vi "rsidr_core_global.vi"() -> ()   [LabVIEW 2020, in "Rohde&Schwarz CMWXP NR FR1 Measurement.lvlib"] (continued)
 "Flags"=0, "Help"="Put a help here"}, {"Level"=3, "Class Only"=FALSE, "Identifier"="RSCMWXPNRFR1M_ATTR_MULTI_EVAL_MEAS_TRIGGER_SOURCE", "Descriptive Name"="Multi Eval Meas Trigger Source", "Data Type"=enum."ViString", "Command"="TRIG:NRS:MEAS{instance}:MEV:SOUR", "Access"=enum."Read/Write", "Range Table"="", "Read Callback"="", "Write Callback"="", "Range Callback"="", "Check Callback"="", "Rngtable Callback"="", "Coerce Callback"="", "Supported Models"="", "Instrument Options"="", "Check Status Callback"="", "Flags"=0, "Help"="Selects the source of the trigger events. Some values are always available. They are listed below. Depending on the installed options, additional values are available. You can query a list of all supported values via TRIGger:...:CATalog:SOURce?.\n\nAvailable Repeated Capabilities:\ninstance: i0, i1, i2, i3, i4, i5, i6, i7, i8, i9, i10, i11, i12, i13, i14, i15, i16, i17, i18, i19, i20, i21, i22, i23, i24, i25, i26, i27, i28, i29, i30, i31, i32\r\n\nRemote-control command(s):\nTRIGger:NRSub:MEAS<i>:MEValuation:SOURce"}, {"Level"=3, "Class Only"=FALSE, "Identifier"="RSCMWXPNRFR1M_ATTR_MULTI_EVAL_MEAS_TRIGGER_SOURCE_CATALOG", "Descriptive Name"="Multi Eval Meas Trigger Source Catalog", "Data Type"=enum."RawString", "Command"="TRIG:NRS:MEAS{instance}:MEV:CAT:SOUR?", "Access"=enum."Read Only", "Range Table"="", "Read Callback"="", "Write Callback"="", "Range Callback"="", "Check Callback"="", "Rngtable Callback"="", "Coerce Callback"="", "Supported Models"="", "Instrument Options"="", "Check Status Callback"="", "Flags"=0, "Help"="Lists all trigger source values that can be set using TRIGger:NRSub:MEAS<i>:MEValuation:SOURce.\n\nAvailable Repeated Capabilities:\ninstance: i0, i1, i2, i3, i4, i5, i6, i7, i8, i9, i10, i11, i12, i13, i14, i15, i16, i17, i18, i19, i20, i21, i22, i23, i24, i25, i26, i27, i28, i29, i30, i31, i32\r\n\nRemote-control command(s):\nTRIGger:NRSub:MEAS<i>:MEValuation:CATalog:SOURce?"}, {"Level"=3, "Class Only"=FALSE, "Identifier"="RSCMWXPNRFR1M_ATTR_MULTI_EVAL_MEAS_TRIGGER_SLOPE", "Descriptive Name"="Multi Eval Meas Trigger Slope", "Data Type"=enum."ViInt32", "Command"="TRIG:NRS:MEAS{instance}:MEV:SLOP", "Access"=enum."Read/Write", "Range Table"="rsCmwxpNrFr1M_rngTrigSlope", "Read Callback"="", "Write Callback"="", "Range Callback"="", "Check Callback"="", "Rngtable Callback"="", "Coerce Callback"="", "Supported Models"="", "Instrument Options"="", "Check Status Callback"="", "Flags"=0, "Help"="Qualifies whether the trigger event is generated at the rising or at the falling edge of the trigger pulse (valid for external and power trigger sources).\n\nAvailable Repeated Capabilities:\ninstance: i0, i1, i2, i3, i4, i5, i6, i7, i8, i9, i10, i11, i12, i13, i14, i15, i16, i17, i18, i19, i20, i21, i22, i23, i24, i25, i26, i27, i28, i29, i30, i31, i32\r\n\nRemote-control command(s):\nTRIGger:NRSub:MEAS<i>:MEValuation:SLOPe"}, {"Level"=3, "Class Only"=FALSE, "Identifier"="RSCMWXPNRFR1M_ATTR_MULTI_EVAL_MEAS_TRIGGER_THRESHOLD", "Descriptive Name"="Multi Eval Meas Trigger Threshold", "Data Type"=enum."ViReal64", "Command"="TRIG:NRS:MEAS{instance}:MEV:THR", "Access"=enum."Read/Write", "Range Table"="rsCmwxpNrFr1M_rngTrigThreshold", "Read Callback"="", "Write Callback"="", "Range Callback"="", "Check Callback"="", "Rngtable Callback"="", "Coerce Callback"="", "Supported Models"="", "Instrument Options"="", "Check Status Callback"="", "Flags"=0, "Help"="Defines the trigger threshold for power trigger sources.\n\nAvailable Repeated Capabilities:\ninstance: i0, i1, i2, i3, i4, i5, i6, i7, i8, i9, i10, i11, i12, i13, i14, i15, i16, i17, i18, i19, i20, i21, i22, i23, i24, i25, i26, i27, i28, i29, i30, i31, i32\r\n\nRemote-control command(s):\nTRIGger:NRSub:MEAS<i>:MEValuation:THReshold"}, {"Level"=3, "Class Only"=FALSE, "Identifier"="RSCMWXPNRFR1M_ATTR_MULTI_EVAL_MEAS_TRIGGER_DELAY", "Descriptive Name"="Multi Eval Meas Trigger Delay", "Data Type"=enum."ViReal64", "Command"="TRIG:NRS:MEAS{instance}:MEV:DEL", "Access"=enum."Read/Write", "Range Table"="rsCmwxpNrFr1M_rngMultiEvalMeasurementTriggerDelay", "Read Callback"="", "Write Callback"="", "Range Callback"="", "Check Callback"="", "Rngtable Callback"="", "Coerce Callback"="", "Supported Models"="", "Instrument Options"="", "Check Status Callback"="", "Flags"=0, "Help"="Defines a time delaying the start of the measurement relative to the trigger event. This setting has no influence on free run measurements.\n\nAvailable Repeated Capabilities:\ninstance: i0, i1, i2, i3, i4, i5, i6, i7, i8, i9, i10, i11, i12, i13, i14, i15, i16, i17, i18, i19, i20, i21, i22, i23, i24, i25, i26, i27, i28, i29, i30, i31, i32\r\n\nRemote-control command(s):\nTRIGger:NRSub:MEAS<i>:MEValuation:DELay"}, {"Level"=3, "Class Only"=FALSE, "Identifier"="RSCMWXPNRFR1M_ATTR_MULTI_EVAL_MEAS_TRIGGER_TIMEOUT_ENABLED", "Descriptive Name"="Multi Eval Meas Trigger Timeout Enabled", "Data Type"=enum."ViBoolean", "Command"="TRIG:NRS:MEAS{instance}:MEV:TOUT", "Access"=enum."Read/Write", "Range Table"="", "Read Callback"="", "Write Callback"="", "Range Callback"="", "Check Callback"="", "Rngtable Callback"="", "Coerce Callback"="", "Supported Models"="", "Instrument Options"="", "Check Status Callback"="", "Flags"=0, "Help"="Selects the maximum time that the measurement waits for a trigger event before it stops in remote control mode or indicates a trigger timeout in manual operation mode. This setting has no influence on Free Run measurements.\n\nAvailable Repeated Capabilities:\ninstance: i0, i1, i2, i3, i4, i5, i6, i7, i8, i9, i10, i11, i12, i13, i14, i15, i16, i17, i18, i19, i20, i21, i22, i23, i24, i25, i26, i27, i28, i29, i30, i31, i32\r\n\nRemote-control command(s):\nTRIGger:NRSub:MEAS<i>:MEValuation:TOUT"}, {"Level"=3, "Class Only"=FALSE, "Identifier"="RSCMWXPNRFR1M_ATTR_MULTI_EVAL_MEAS_TRIGGER_TIMEOUT", "Descriptive Name"="Multi Eval Meas Trigger Timeout", "Data Type"=enum."ViReal64", "Command"="TRIG:NRS:MEAS{instance}:MEV:TOUT", "Access"=enum."Read/Write", "Range Table"="rsCmwxpNrFr1M_rngTriggerTimeout", "Read Callback"="", "Write Callback"="", "Range Callback"="", "Check Callback"="", "Rngtable Callback"="", "Coerce Callback"="", "Supported Models"="", "Instrument Options"="", "Check Status Callback"="", "Flags"=0, "Help"="Selects the maximum time that the measurement waits for a trigger event before it stops in remote control mode or indicates a trigger timeout in manual operation mode. This setting has no influence on Free Run measurements.\n\nAvailable Repeated Capabilities:\ninstance: i0, i1, i2, i3, i4, i5, i6, i7, i8, i9, i10, i11, i12, i13, i14, i15, i16, i17, i18, i19, i20, i21, i22, i23, i24, i25, i26, i27, i28, i29, i30, i31, i32\r\n\nRemote-control command(s):\nTRIGger:NRSub:MEAS<i>:MEValuation:TOUT"}, {"Level"=3, "Class Only"=FALSE, "Identifier"="RSCMWXPNRFR1M_ATTR_MULTI_EVAL_MEAS_MINIMUM_TRIGGER_GAP", "Descriptive Name"="Multi Eval Meas Minimum Trigger Gap", "Data Type"=enum."ViReal64", "Command"="TRIG:NRS:MEAS{instance}:MEV:MGAP", "Access"=enum."Read/Write", "Range Table"="rsCmwxpNrFr1M_rngMinimumTriggerGap", "Read Callback"="", "Write Callback"="", "Range Callback"="", "Check Callback"="", "Rngtable Callback"="", "Coerce Callback"="", "Supported Models"="", "Instrument Options"="", "Check Status Callback"="", "Flags"=0, "Help"="Sets a minimum time during which the IF signal must be below the trigger threshold before the trigger is armed so that an IF power trigger event can be generated.\n\nAvailable Repeated Capabilities:\ninstance: i0, i1, i2, i3, i4, i5, i6, i7, i8, i9, i10, i11, i12, i13, i14, i15, i16, i17, i18, i19, i20, i21, i22, i23, i24, i25, i26, i27, i28, i29, i30, i31, i32\r\n\nRemote-control command(s):\nTRIGger:NRSub:MEAS<i>:MEValuation:MGAP"}, {"Level"=3, "Class Only"=FALSE, "Identifier"="RSCMWXPNRFR1M_ATTR_MULTI_EVAL_MEAS_TRIGGER_SYNC_MODE", "Descriptive Name"="Multi Eval Meas Trigger Sync Mode", "Data Type"=enum."ViInt32", "Command"="TRIG:NRS:MEAS{instance}:MEV:SMOD", "Access"=enum."Read/Write", "Range Table"="rsCmwxpNrFr1M_rngTriggerSyncMode", "Read Callback"="", "Write Callback"="", "Range Callback"="", "Check Callback"="", "Rngtable Callback"="", "Coerce Callback"="", "Supported Models"="", "Instrument Options"="", "Check Status Callback"="", "Flags"=0, "Help"="Selects the size of the search window for synchronization - normal or enhanced.\n\nAvailable Repeated Capabilities:\ninstance: i0, i1, i2, i3, i4, i5, i6, i7, i8, i9, i10, i11, i12, i13, i14, i15, i16, i17, i18, i19, i20, i21, i22, i23, i24, i25, i26, i27, i28, i29, i30, i31, i32\r\n\nRemote-control command(s):\nTRIGger:NRSub:MEAS<i>:MEValuation:SMODe"}, {"Level"=3, "Class Only"=FALSE, "Identifier"="RSCMWXPNRFR1M_ATTR_MULTI_EVAL_MEAS_TRIGGER_LIST_MODE", "Descriptive Name"="Multi Eval Meas Trigger List Mode", "Data Type"=enum."ViInt32", "Command"="TRIG:NRS:MEAS{instance}:MEV:LIST:MODE", "Access"=enum."Read/Write", "Range Table"="rsCmwxpNrFr1M_rngTriggerListMode", "Read Callback"="", "Write Callback"="", "Range Callback"="", "Check Callback"="", "Rngtable Callback"="", "Coerce Callback"="", "Supported Models"="", "Instrument Options"="", "Check Status Callback"="", "Flags"=0, "Help"="Specifies the trigger mode for list mode measurements. For configuration of retrigger flags, see CONFigure:NRSub:MEAS<i>:LIST:SEGMent<no>:SETup.\n\nAvailable Repeated Capabilities:\ninstance: i0, i1, i2, i3, i4, i5, i6, i7, i8, i9, i10, i11, i12, i13, i14, i15, i16, i17, i18, i19, i20, i21, i22, i23, i24, i25, i26, i27, i28, i29, i30, i31, i32\r\n\nRemote-control command(s):\nTRIGger:NRSub:MEAS<i>:MEValuation:LIST:MODE"}, {"Level"=2, "Class Only"=TRUE, "Identifier"="", "Descriptive Name"="Limits", "Data Type"=enum."ViInt32", "Command"="", "Access"=enum."Read Only", "Range Table"="", "Read Callback"="", "Write Callback"="", "Range Callback"="", "Check Callback"="", "Rngtable Callback"="", "Coerce Callback"="", "Supported Models"="", "Instrument Options"="", "Check Status Callback"="", "Flags"=0, "Help"="Multi Evaluation measurement limits attributes."}, {"Level"=3, "Class Only"=TRUE, "Identifier"="", "Descriptive Name"="Modulation", "Data Type"=enum."ViInt32", "Command"="", "Access"=enum."Read Only", "Range Table"="", "Read Callback"="", "Write Callback"="", "Range Callback"="", "Check Callback"="", "Rngtable Callback"="", "Coerce Callback"="", "Supported Models"="", "Instrument Options"="", "Check Status Callback"="", "Flags"=0, "Help"="Contains attributes for selected modulation."}, {"Level"=4, "Class Only"=TRUE, "Identifier"="", "Descriptive Name"="Pi/2-BPSK", "Data Type"=enum."ViInt32", "Command"="", "Access"=enum."Read Only", "Range Table"="", "Read Callback"="", "Write Callback"="", "Range Callback"="", "Check Callback"="", "Rngtable Callback"="", "Coerce Callback"="", "Supported Models"="", "Instrument Options"="", "Check Status Callback"="", "Flags"=0, "Help"="Define limits for results which characterize the modulation accuracy of signals with modulation scheme Pi/2-BPSK."}, {"Level"=5, "Class Only"=FALSE, "Identifier"="RSCMWXPNRFR1M_ATTR_MULTI_EVAL_MEAS_LIMIT_PI_2_EVM", "Descriptive Name"="Multi Eval Meas Limit Pi/2 BPSK EVM", "Data Type"=enum."RawString", "Command"="CONF:NRS:MEAS{instance}:MEV:LIM:PHBP:EVM", "Access"=enum."Read/Write", "Range Table"="", "Read Callback"="", "Write Callback"="", "Range Callback"="", "Check Callback"="", "Rngtable Callback"="", "Coerce Callback"="", "Supported Models"="", "Instrument Options"="", "Check Status Callback"="", "Flags"=0, "Help"="Defines upper limits for the RMS and peak values of the error vector magnitude (EVM) for Pi/2-BPSK.\n\nSyntax:\nCONFigure:NRSub:MEAS<i>:MEValuation:LIMit:PHBPsk:EVMagnitude <RMS>, <Peak>\n\n<RMS>\nnumeric | ON | OFF\nValid Values:\n0 % to 100 %\n  \n<Peak>\nnumeric | ON | OFF\nValid Values:\n0 % to 100 %\n\nAvailable Repeated Capabilities:\ninstance: i0, i1, i2, i3, i4, i5, i6, i7, i8, i9, i10, i11, i12, i13, i14, i15, i16, i17, i18, i19, i20, i21, i22, i23, i24, i25, i26, i27, i28, i29, i30, i31, i32\r\n\nRemote-control command(s):\nCONFigure:NRSub:MEAS<i>:MEValuation:LIMit:PHBPsk:EVMagnitude"}, {"Level"=5, "Class Only"=FALSE, "Identifier"="RSCMWXPNRFR1M_ATTR_MULTI_EVAL_MEAS_LIMIT_PI_2_MERR", "Descriptive Name"="Multi Eval Meas Limit Pi/2 BPSK MERR", "Data Type"=enum."RawString", "Command"="CONF:NRS:MEAS{instance}:MEV:LIM:PHBP:MERR", "Access"=enum."Read/Write", "Range Table"="", "Read Callback"="", "Write Callback"="", "Range Callback"="", "Check Callback"="", "Rngtable Callback"="", "Coerce Callback"="", "Supported Models"="", "Instrument Options"="", "Check Status Callback"="", "Flags"=0, "Help"="Defines upper limits for the RMS and peak values of the magnitude error for Pi/2-BPSK.\n\nSyntax:\nCONFigure:NRSub:MEAS<i>:MEValuation:LIMit:PHBPsk:MERRor <RMS>, <Peak>\n\n<RMS>\nnumeric | ON | OFF\nValid Values:\n0 % to 100 %\n  \n<Peak>\nnumeric | ON | OFF\nValid Values:\n0 % to 100 %\n\nAvailable Repeated Capabilities:\ninstance: i0, i1, i2, i3, i4, i5, i6, i7, i8, i9, i10, i11, i12, i13, i14, i15, i16, i17, i18, i19, i20, i21, i22, i23, i24, i25, i26, i27, i28, i29, i30, i31, i32\r\n\nRemote-control command(s):\nCONFigure:NRSub:MEAS<i>:MEValuation:LIMit:PHBPsk:MERRor"}, {"Level"=5, "Class Only"=FALSE, "Identifier"="RSCMWXPNRFR1M_ATTR_MULTI_EVAL_MEAS_LIMIT_PI_2_PERR", "Descriptive Name"="Multi Eval Meas Limit Pi/2 BPSK PERR", "Data Type"=enum."RawString", "Command"="CONF:NRS:MEAS{instance}:MEV:LIM:PHBP:PERR", "Access"=enum."Read/Write", "Range Table"="", "Read Callback"="", "Write Callback"="", "Range Callback"="", "Check Callback"="", "Rngtable Callback"="", "Coerce Callback"="", "Supported Models"="", "Instrument Options"="", "Check Status Callback"="", "Flags"=0, "Help"="Defines symmetric limits for the RMS and peak values of the phase error for Pi/2-BPSK. The limit check fails if the absolute value of the measured phase error exceeds the specified values.\n\nSyntax:\nCONFigure:NRSub:MEAS<i>:MEValuation:LIMit:PHBPsk:PERRor <RMS>, <Peak>\n\n<RMS>\nnumeric | ON | OFF\nValid Values:\n0 deg to 180 deg\n  \n<Peak>\nnumeric | ON | OFF\nValid Values:\n0 deg to 180 deg\n\nAvailable Repeated Capabilities:\ninstance: i0, i1, i2, i3, i4, i5, i6, i7, i8, i9, i10, i11, i12, i13, i14, i15, i16, i17, i18, i19, i20, i21, i22, i23, i24, i25, i26, i27, i28, i29, i30, i31, i32\r\n\nRemote-control command(s):\nCONFigure:NRSub:MEAS<i>:MEValuation:LIMit:PHBPsk:PERRor"}, {"Level"=5, "Class Only"=FALSE, "Identifier"="RSCMWXPNRFR1M_ATTR_MULTI_EVAL_MEAS_LIMIT_PI_2_FERR_ENABLED", "Descriptive Name"="Multi Eval Meas Limit Pi/2 BPSK FERR Enabled", "Data Type"=enum."ViBoolean", "Command"="CONF:NRS:MEAS{instance}:MEV:LIM:PHBP:FERR", "Access"=enum."Read/Write", "Range Table"="", "Read Callback"="", "Write Callback"="", "Range Callback"="", "Check Callback"="", "Rngtable Callback"="", "Coerce Callback"="", "Supported Models"="", "Instrument Options"="", "Check Status Callback"="", "Flags"=0, "Help"="Defines an upper limit for the carrier frequency error (Pi/2-BPSK modulation).\n\nAvailable Repeated Capabilities:\ninstance: i0, i1, i2, i3, i4, i5, i6, i7, i8, i9, i10, i11, i12, i13, i14, i15, i16, i17, i18, i19, i20, i21, i22, i23, i24, i25, i26, i27, i28, i29, i30, i31, i32\r\n\nRemote-control command(s):\nCONFigure:NRSub:MEAS<i>:MEValuation:LIMit:PHBPsk:FERRor"}, {"Level"=5, "Class Only"=FALSE, "Identifier"="RSCMWXPNRFR1M_ATTR_MULTI_EVAL_MEAS_LIMIT_PI_2_FERR", "Descriptive Name"="Multi Eval Meas Limit Pi/2 BPSK FERR", "Data Type"=enum."ViReal64", "Command"="CONF:NRS:MEAS{instance}:MEV:LIM:PHBP:FERR", "Access"=enum."Read/Write", "Range Table"="rsCmwxpNrFr1M_rngFERR", "Read Callback"="", "Write Callback"="", "Range Callback"="", "Check Callback"="", "Rngtable Callback"="", "Coerce Callback"="", "Supported Models"="", "Instrument Options"="", "Check Status Callback"="", "Flags"=0, "Help"="Defines an upper limit for the carrier frequency error (Pi/2-BPSK modulation).\n\nAvailable Repeated Capabilities:\ninstance: i0, i1, i2, i3, i4, i5, i6, i7, i8, i9, i10, i11, i12, i13, i14, i15, i16, i17, i18, i19, i20, i21, i22, i23, i24, i25, i26, i27, i28, i29, i30, i31, i32\r\n\nRemote-control command(s):\nCONFigure:NRSub:MEAS<i>:MEValuation:LIMit:PHBPsk:FERRor"}, {"Level"=5, "Class Only"=FALSE, "Identifier"="RSCMWXPNRFR1M_ATTR_MULTI_EVAL_MEAS_LIMIT_PI_2_IQ_OFFSET", "Descriptive Name"="Multi Eval Meas Limit Pi/2 BPSK IQ Offset", "Data Type"=enum."RawString", "Command"="CONF:NRS:MEAS{instance}:MEV:LIM:PHBP:IQOF", "Access"=enum."Read/Write", "Range Table"="", "Read Callback"="", "Write Callback"="", "Range Callback"="", "Check Callback"="", "Rngtable Callback"="", "Coerce Callback"="", "Supported Models"="", "Instrument Options"="", "Check Status Callback"="", "Flags"=0, "Help"="Defines upper limits for the I/Q origin offset (Pi/2-BPSK modulation). Four different I/Q origin offset limits can be set for four TX power ranges.\n\nSyntax:\nCONFigure:NRSub:MEAS<i>:MEValuation:LIMit:PHBPsk:IQOFfset <Enable>, <Offset0>, <Offset1>,<Offset2>,<Offset3>\n\n<Enable>\nValid Values:\nOFF: disables the limit check\nON: enables the limit check\n\n<Offset0>\nI/Q origin offset limit for TX power > 10 dBm\nnumeric\nValid Values: -256 dBc to 256 dBc\n\n<Offset1>\nI/Q origin offset limit for TX power > 0 dBm\nnumeric\nValid Values: -256 dBc to 256 dBc\n\n<Offset2>\nI/Q origin offset limit for TX power > -30 dBm\nnumeric\nValid Values: -256 dBc to 256 dBc\n\n<Offset3>\nI/Q origin offset limit for TX power > -40 dBm\nnumeric\nValid Values: -256 dBc to 256 dBc\n\nAvailable Repeated Capabilities:\ninstance: i0, i1, i2, i3, i4, i5, i6, i7, i8, i9, i10, i11, i12, i13, i14, i15, i16, i17, i18, i19, i20, i21, i22, i23, i24, i25, i26, i27, i28, i29, i30, i31, i32\r\n\nRemote-control command(s):\nCONFigure:NRSub:MEAS<i>:MEValuation:LIMit:PHBPsk:IQOFfset"}, {"Level"=5, "Class Only"=FALSE, "Identifier"="RSCMWXPNRFR1M_ATTR_MULTI_EVAL_MEAS_LIMIT_PI_2_INBAND_EMISSION", "Descriptive Name"="Multi Eval Meas Limit Pi/2 BPSK Inband Emission", "Data Type"=enum."RawString", "Command"="CONF:NRS:MEAS{instance}:MEV:LIM:PHBP:IBE", "Access"=enum."Read/Write", "Range Table"="", "Read Callback"="", "Write Callback"="", "Range Callback"="", "Check Callback"="", "Rngtable Callback"="", "Coerce Callback"="", "Supported Models"="", "Instrument Options"="", "Check Status Callback"="", "Flags"=0, "Help"="Defines parameters used for calculation of an upper limit for the inband emission (Pi/2-BPSK modulation), see 'Inband Emissions Limits'.\n\nSyntax:\nCONFigure:NRSub:MEAS<i>:MEValuation:LIMit:PHBPsk:IBE <Enable>, <Minimum>, <EVM>, <RBPower>, <IQImageLesser>, <IQImageGreater>\n\n<Enable>\nValid Values:\nOFF: disables the limit check\nON: enables the limit check\n\n<Minimum>\nnumeric\nValid Values: -256 dB to 256 dB\n\n<EVM>\nnumeric\nValid Values: 0 % to 100 %\n\n<RBPower>\nnumeric\nValid Values: -256 dBm to 256 dBm\n\n<IQImageLesser>\nIQ image for low TX power range\nnumeric\nValid Values: -256 dB to 256 dB\n \n<IQImageGreater>\nIQ image for high TX power range\nnumeric\nValid Values: -256 dB  to  256 dB\n\nAvailable Repeated Capabilities:\ninstance: i0, i1, i2, i3, i4, i5, i6, i7, i8, i9, i10, i11, i12, i13, i14, i15, i16, i17, i18, i19, i20, i21, i22, i23, i24, i25, i26, i27, i28, i29, i30, i31, i32\r\n\nRemote-control command(s):\nCONFigure:NRSub:MEAS<i>:MEValuation:LIMit:PHBPsk:IBE"}, {"Level"=5, "Class Only"=FALSE, "Identifier"="RSCMWXPNRFR1M_ATTR_MULTI_EVAL_MEAS_LIMIT_PI_2_INBAND_EMISSION_IQ_OFFSET", "Descriptive Name"="Multi Eval Meas Limit Pi/2 BPSK Inband Emission IQ Offset", "Data Type"=enum."RawString", "Command"="CONF:NRS:MEAS{instance}:MEV:LIM:PHBP:IBE:IQOF", "Access"=enum."Read/Write", "Range Table"="", "Read Callback"="", "Write Callback"="", "Range Callback"="", "Check Callback"="", "Rngtable Callback"="", "Coerce Callback"="", "Supported Models"="", "Instrument Options"="", "Check Status Callback"="", "Flags"=0, "Help"="Defines I/Q origin offset values used for calculation of an upper limit for the inband emission, for Pi/2-BPSK modulation. Four different values can be set for four TX power ranges.\n\nSyntax:\nCONFigure:NRSub:MEAS<i>:MEValuation:LIMit:PHBPsk:IBE:IQOFfset <Offset0>, <Offset1>,<Offset2>,<Offset3>\n\n<Offset0>\nI/Q origin offset limit for TX power > 10 dBm\nnumeric\nValid Values: -256 dBc to 256 dBc\n\n<Offset1>\nI/Q origin offset limit for TX power > 0 dBm\nnumeric\nValid Values: -256 dBc to 256 dBc\n\n<Offset2>\nI/Q origin offset limit for TX power > -30 dBm\nnumeric\nValid Values: -256 dBc to 256 dBc\n\n<Offset3>\nI/Q origin offset limit for TX power > -40 dBm\nnumeric\nValid Values: -256 dBc to 256 dBc\n\nAvailable Repeated Capabilities:\ninstance: i0, i1, i2, i3, i4, i5, i6, i7, i8, i9, i10, i11, i12, i13, i14, i15, i16, i17, i18, i19, i20, i21, i22, i23, i24, i25, i26, i27, i28, i29, i30, i31, i32\r\n\nRemote-control command(s):\nCONFigure:NRSub:MEAS<i>:MEValuation:LIMit:PHBPsk:IBE:IQOFfset"}, {"Level"=5, "Class Only"=FALSE, "Identifier"="RSCMWXPNRFR1M_ATTR_MULTI_EVAL_MEAS_LIMIT_PI_2_EQUALIZER_SPECTRUM_FLATNESS", "Descriptive Name"="Multi Eval Meas Limit Pi/2 BPSK Equalizer Spectrum Flatness", "Data Type"=enum."RawString", "Command"="CONF:NRS:MEAS{instance}:MEV:LIM:PHBP:ESFL", "Access"=enum."Read/Write", "Range Table"="", "Read Callback"="", "Write Callback"="", "Range Callback"="", "Check Callback"="", "Rngtable Callback"="", "Coerce Callback"="", "Supported Models"="", "Instrument Options"="", "Check Status Callback"="", "Flags"=0, "Help"="Defines limits for the equalizer spectrum flatness (Pi/2-BPSK modulation).\n\nSyntax:\nCONFigure:NRSub:MEAS<i>:MEValuation:LIMit:PHBPsk:ESFLatness <Enable>, <Range1>, <Range2>, <Max1Min2>, <Max2Min1>, <EdgeFrequency>\n\n<Enable>\nValid Values:\nOFF: disables the limit check\nON: enables the limit check\n\n<Range1>\nUpper limit for max(range 1) - min(range 1)\nnumeric\nValid Values: -256 dBpp to 256 dBpp \n\n<Range2>\nUpper limit for max(range 2) - min(range 2)\nnumeric\nValid Values: -256 dBpp to 256 dBpp \n\n<Max1Min2>\nUpper limit for max(range 1) - min(range 2)\nnumeric\nValid Values: -256 dB to 256 dB \n\n<Max2Min1>\nUpper limit for max(range 2) - min(range 1)\nnumeric\nValid Values: -256 dB to 256 dB\n\n<EdgeFrequency>\nBand edge distance of border between range 1 and range 2\nValid Values:\n0 MHz to 20 MHz\n\nAvailable Repeated Capabilities:\ninstance: i0, i1, i2, i3, i4, i5, i6, i7, i8, i9, i10, i11, i12, i13, i14, i15, i16, i17, i18, i19, i20, i21, i22, i23, i24, i25, i26, i27, i28, i29, i30, i31, i32\r\n\nRemote-control command(s):\nCONFigure:NRSub:MEAS<i>:MEValuation:LIMit:PHBPsk:ESFLatness"}, {"Level"=4, "Class Only"=TRUE, "Identifier"="", "Descriptive Name"="BPSK Shaping", "Data Type"=enum."ViInt32", "Command"="", "Access"=enum."Read Only", "Range Table"="", "Read Callback"="", "Write Callback"="", "Range Callback"="", "Check Callback"="", "Rngtable Callback"="", "Coerce Callback"="", "Supported Models"="", "Instrument Options"="", "Check Status Callback"="", "Flags"=0, "Help"="Define limits for results which characterize the modulation accuracy of signals with modulation scheme BPSK Shaping."}, {"Level"=5, "Class Only"=FALSE, "Identifier"="RSCMWXPNRFR1M_ATTR_MULTI_EVAL_MEAS_LIMIT_BPSK_SHAPING_EVM", "Descriptive Name"="Multi Eval Meas Limit BPSK Shaping EVM", "Data Type"=enum."RawString", "Command"="CONF:NRS:MEAS{instance}:MEV:LIM:BPWS:EVM", "Access"=enum."Read/Write", "Range Table"="", "Read Callback"="", "Write Callback"="", "Range Callback"="", "Check Callback"="", "Rngtable Callback"="", "Coerce Callback"="", "Supported Models"="", "Instrument Options"="", "Check Status Callback"="", "Flags"=0, "Help"="Defines upper limits for the RMS and peak values of the error vector magnitude (EVM) for /2-BPSK with shaping.\n\nSyntax:\nCONFigure:NRSub:MEAS<i>:MEValuation:LIMit:BPWShaping:EVMagnitude <RMS>, <Peak>\n\n<RMS>\nnumeric | ON | OFF\nValid Values:\n0 % to 100 %\n  \n<Peak>\nnumeric | ON | OFF\nValid Values:\n0 % to 100 %\n\nAvailable Repeated Capabilities:\ninstance: i0, i1, i2, i3, i4, i5, i6, i7, i8, i9, i10, i11, i12, i13, i14, i15, i16, i17, i18, i19, i20, i21, i22, i23, i24, i25, i26, i27, i28, i29, i30, i31, i32\r\n\nRemote-control command(s):\nCONFigure:NRSub:MEAS<i>:MEValuation:LIMit:BPWShaping:EVMagnitude"}, {"Level"=5, "Class Only"=FALSE, "Identifier"="RSCMWXPNRFR1M_ATTR_MULTI_EVAL_MEAS_LIMIT_BPSK_SHAPING_MERR", "Descriptive Name"="Multi Eval Meas Limit BPSK Shaping MERR", "Data Type"=enum."RawString", "Command"="CONF:NRS:MEAS{instance}:MEV:LIM:BPWS:MERR", "Access"=enum."Read/Write", "Range Table"="", "Read Callback"="", "Write Callback"="", "Range Callback"="", "Check Callback"="", "Rngtable Callback"="", "Coerce Callback"="", "Supported Models"="", "Instrument Options"="", "Check Status Callback"="", "Flags"=0, "Help"="Defines upper limits for the RMS and peak values of the magnitude error for /2-BPSK with shaping.\n\nSyntax:\nCONFigure:NRSub:MEAS<i>:MEValuation:LIMit:PHBPsk:MERRor <RMS>, <Peak>\n\n<RMS>\nnumeric | ON | OFF\nValid Values:\n0 % to 100 %\n  \n<Peak>\nnumeric | ON | OFF\nValid Values:\n0 % to 100 %\n\nAvailable Repeated Capabilities:\ninstance: i0, i1, i2, i3, i4, i5, i6, i7, i8, i9, i10, i11, i12, i13, i14, i15, i16, i17, i18, i19, i20, i21, i22, i23, i24, i25, i26, i27, i28, i29, i30, i31, i32\r\n\nRemote-control command(s):\nCONFigure:NRSub:MEAS<i>:MEValuation:LIMit:BPWShaping:MERRor"}, {"Level"=5, "Class Only"=FALSE, "Identifier"="RSCMWXPNRFR1M_ATTR_MULTI_EVAL_MEAS_LIMIT_BPSK_SHAPING_PERR", "Descriptive Name"="Multi Eval Meas Limit BPSK Shaping PERR", "Data Type"=enum."RawString", "Command"="CONF:NRS:MEAS{instance}:MEV:LIM:BPWS:PERR", "Access"=enum."Read/Write", "Range Table"="", "Read Callback"="", "Write Callback"="", "Range Callback"="", "Check Callback"="", "Rngtable Callback"="", "Coerce Callback"="", "Supported Models"="", "Instrument Options"="", "Check Status Callback"="", "Flags"=0, "Help"="Defines symmetric limits for the RMS and peak values of the phase error for /2-BPSK with shaping. The limit check fails if the absolute value of the measured phase error exceeds the specified values.\n\nSyntax:\nCONFigure:NRSub:MEAS<i>:MEValuation:LIMit:BPWShaping:PERRor <RMS>, <Peak>\n\n<RMS>\nnumeric | ON | OFF\nValid Values:\n0 deg to 180 deg\n  \n<Peak>\nnumeric | ON | OFF\nValid Values:\n0 deg to 180 deg\n\nAvailable Repeated Capabilities:\ninstance: i0, i1, i2, i3, i4, i5, i6, i7, i8, i9, i10, i11, i12, i13, i14, i15, i16, i17, i18, i19, i20, i21, i22, i23, i24, i25, i26, i27, i28, i29, i30, i31, i32\r\n\nRemote-control command(s):\nCONFigure:NRSub:MEAS<i>:MEValuation:LIMit:BPWShaping:PERRor"}, {"Level"=5, "Class Only"=FALSE, "Identifier"="RSCMWXPNRFR1M_ATTR_MULTI_EVAL_MEAS_LIMIT_BPSK_SHAPING_FERR_ENABLED", "Descriptive Name"="Multi Eval Meas Limit BPSK Shaping FERR Enabled", "Data Type"=enum."ViBoolean", "Command"="CONF:NRS:MEAS{instance}:MEV:LIM:BPWS:FERR", "Access"=enum."Read/Write", "Range Table"="", "Read Callback"="", "Write Callback"="", "Range Callback"="", "Check Callback"="", "Rngtable Callback"="", "Coerce Callback"="", "Supported Models"="", "Instrument Options"="", "Check Status Callback"="", "Flags"=0, "Help"="Defines an upper limit for the carrier frequency error (/2-BPSK modulation with shaping).\n\nAvailable Repeated Capabilities:\ninstance: i0, i1, i2, i3, i4, i5, i6, i7, i8, i9, i10, i11, i12, i13, i14, i15, i16, i17, i18, i19, i20, i21, i22, i23, i24, i25, i26, i27, i28, i29, i30, i31, i32\r\n\nRemote-control command(s):\nCONFigure:NRSub:MEAS<i>:MEValuation:LIMit:BPWShaping:FERRor"}, {"Level"=5, "Class Only"=FALSE, "Identifier"="RSCMWXPNRFR1M_ATTR_MULTI_EVAL_MEAS_LIMIT_BPSK_SHAPING_FERR", "Descriptive Name"="Multi Eval Meas Limit BPSK Shaping FERR", "Data Type"=enum."ViReal64", "Command"="CONF:NRS:MEAS{instance}:MEV:LIM:BPWS:FERR", "Access"=enum."Read/Write", "Range Table"="rsCmwxpNrFr1M_rngFERR", "Read Callback"="", "Write Callback"="", "Range Callback"="", "Check Callback"="", "Rngtable Callback"="", "Coerce Callback"="", "Supported Models"="", "Instrument Options"="", "Check Status Callback"="", "Flags"=0, "Help"="Defines an upper limit for the carrier frequency error (/2-BPSK modulation with shaping).\n\nAvailable Repeated Capabilities:\ninstance: i0, i1, i2, i3, i4, i5, i6, i7, i8, i9, i10, i11, i12, i13, i14, i15, i16, i17, i18, i19, i20, i21, i22, i23, i24, i25, i26, i27, i28, i29, i30, i31, i32\r\n\nRemote-control command(s):\nCONFigure:NRSub:MEAS<i>:MEValuation:LIMit:BPWShaping:FERRor"}, {"Level"=5, "Class Only"=FALSE, "Identifier"="RSCMWXPNRFR1M_ATTR_MULTI_EVAL_MEAS_LIMIT_BPSK_SHAPING_IQ_OFFSET", "Descriptive Name"="Multi Eval Meas Limit BPSK Shaping IQ Offset", "Data Type"=enum."RawString", "Command"="CONF:NRS:MEAS{instance}:MEV:LIM:BPWS:IQOF", "Access"=enum."Read/Write", "Range Table"="", "Read Callback"="", "Write Callback"="", "Range Callback"="", "Check Callback"="", "Rngtable Callback"="", "Coerce Callback"="", "Supported Models"="", "Instrument Options"="", "Check Status Callback"="", "Flags"=0, "Help"="Defines upper limits for the I/Q origin offset (/2-BPSK modulation with shaping). Four different I/Q origin offset limits can be set for four TX power ranges.\n\nSyntax:\nCONFigure:NRSub:MEAS<i>:MEValuation:LIMit:BPWShaping:IQOFfset <Enable>, <Offset0>, <Offset1>,<Offset2>,<Offset3>\n\n<Enable>\nValid Values:\nOFF: disables the limit check\nON: enables the limit check\n\n<Offset0>\nI/Q origin offset limit for TX power > 10 dBm\nnumeric\nValid Values: -256 dBc to 256 dBc\n\n<Offset1>\nI/Q origin offset limit for TX power > 0 dBm\nnumeric\nValid Values: -256 dBc to 256 dBc\n\n<Offset2>\nI/Q origin offset limit for TX power > -30 dBm\nnumeric\nValid Values: -256 dBc to 256 dBc\n\n<Offset3>\nI/Q origin offset limit for TX power > -40 dBm\nnumeric\nValid Values: -256 dBc to 256 dBc\n\nAvailable Repeated Capabilities:\ninstance: i0, i1, i2, i3, i4, i5, i6, i7, i8, i9, i10, i11, i12, i13, i14, i15, i16, i17, i18, i19, i20, i21, i22, i23, i24, i25, i26, i27, i28, i29, i30, i31, i32\r\n\nRemote-control command(s):\nCONFigure:NRSub:MEAS<i>:MEValuation:LIMit:BPWShaping:IQOFfset"}, {"Level"=5, "Class Only"=FALSE, "Identifier"="RSCMWXPNRFR1M_ATTR_MULTI_EVAL_MEAS_LIMIT_BPSK_SHAPING_INBAND_EMISSION", "Descriptive Name"="Multi Eval Meas Limit BPSK Shaping Inband Emission", "Data Type"=enum."RawString", "Command"="CONF:NRS:MEAS{instance}:MEV:LIM:BPWS:IBE", "Access"=enum."Read/Write", "Range Table"="", "Read Callback"="", "Write Callback"="", "Range Callback"="", "Check Callback"="", "Rngtable Callback"="", "Coerce Callback"="", "Supported Models"="", "Instrument Options"="", "Check Status Callback"="", "Flags"=0, "Help"="Defines parameters used for calculation of an upper limit for the inband emission (/2-BPSK modulation with shaping), see 'Inband Emissions Limits'.\n\nSyntax:\nCONFigure:NRSub:MEAS<i>:MEValuation:LIMit:BPWShaping:IBE <Enable>, <Minimum>, <EVM>, <RBPower>, <IQImageLesser>, <IQImageGreater>\n\n<Enable>\nValid Values:\nOFF: disables the limit check\nON: enables the limit check\n\n<Minimum>\nnumeric\nValid Values: -256 dB to 256 dB\n\n<EVM>\nnumeric\nValid Values: 0 % to 100 %\n\n<RBPower>\nnumeric\nValid Values: -256 dBm to 256 dBm\n\n<IQImageLesser>\nIQ image for low TX power range\nnumeric\nValid Values: -256 dB to 256 dB\n \n<IQImageGreater>\nIQ image for high TX power range\nnumeric\nValid Values: -256 dB  to  256 dB\n\nAvailable Repeated Capabilities:\ninstance: i0, i1, i2, i3, i4, i5, i6, i7, i8, i9, i10, i11, i12, i13, i14, i15, i16, i17, i18, i19, i20, i21, i22, i23, i24, i25, i26, i27, i28, i29, i30, i31, i32\r\n\nRemote-control command(s):\nCONFigure:NRSub:MEAS<i>:MEValuation:LIMit:BPWShaping:IBE"}, {"Level"=5, "Class Only"=FALSE, "Identifier"="RSCMWXPNRFR1M_ATTR_MULTI_EVAL_MEAS_LIMIT_BPSK_SHAPING_INBAND_EMISSION_IQ_OFFSET", "Descriptive Name"="Multi Eval Meas Limit BPSK Shaping Inband Emission IQ Offset", "Data Type"=enum."RawString", "Command"="CONF:NRS:MEAS{instance}:MEV:LIM:BPWS:IBE:IQOF", "Access"=enum."Read/Write", "Range Table"="", "Read Callback"="", "Write Callback"="", "Range Callback"="", "Check Callback"="", "Rngtable Callback"="", "Coerce Callback"="", "Supported Models"="", "Instrument Options"="", "Check Status Callback"="", "Flags"=0, "Help"="Defines I/Q origin offset values used for calculation of an upper limit for the inband emission, for /2-BPSK modulation with shaping. Four different values can be set for four TX power ranges.\n\nSyntax:\nCONFigure:NRSub:MEAS<i>:MEValuation:LIMit:BPWShaping:IBE:IQOFfset <Offset0>, <Offset1>,<Offset2>,<Offset3>\n\n<Offset0>\nI/Q origin offset limit for TX power > 10 dBm\nnumeric\nValid Values: -256 dBc to 256 dBc\n\n<Offset1>\nI/Q origin offset limit for TX power > 0 dBm\nnumeric\nValid Values: -256 dBc to 256 dBc\n\n<Offset2>\nI/Q origin offset limit for TX power > -30 dBm\nnumeric\nValid Values: -256 dBc to 256 dBc\n\n<Offset3>\nI/Q origin offset limit for TX power > -40 dBm\nnumeric\nValid Values: -256 dBc to 256 dBc\n\nAvailable Repeated Capabilities:\ninstance: i0, i1, i2, i3, i4, i5, i6, i7, i8, i9, i10, i11, i12, i13, i14, i15, i16, i17, i18, i19, i20, i21, i22, i23, i24, i25, i26, i27, i28, i29, i30, i31, i32\r\n\nRemote-control command(s):\nCONFigure:NRSub:MEAS<i>:MEValuation:LIMit:BPWShaping:IBE:IQOFfset"}, {"Level"=5, "Class Only"=FALSE, "Identifier"="RSCMWXPNRFR1M_ATTR_MULTI_EVAL_MEAS_LIMIT_BPSK_SHAPING_EQUALIZER_SPECTRUM_FLATNESS", "Descriptive Name"="Multi Eval Meas Limit BPSK Shaping Equalizer Spectrum Flatness", "Data Type"=enum."RawString", "Command"="CONF:NRS:MEAS{instance}:MEV:LIM:BPWS:ESFL", "Access"=enum."Read/Write", "Range Table"="", "Read Callback"="", "Write Callback"="", "Range Callback"="", "Check Callback"="", "Rngtable Callback"="", "Coerce Callback"="", "Supported Models"="", "Instrument Options"="", "Check Status Callback"="", "Flags"=0, "Help"="Defines limits for the equalizer spectrum flatness (/2-BPSK modulation with shaping).\n\nSyntax:\nCONFigure:NRSub:MEAS<i>:MEValuation:LIMit:BPWShaping:ESFLatness <Enable>, <Range1>, <Range2> <EdgeFrequency>\n\n<Enable>\nValid Values:\nOFF: disables the limit check\nON: enables the limit check\n\n<Range1>\nUpper limit for max(range 1) - min(range 1)\nnumeric\nValid Values: -256 dBpp to 256 dBpp \n\n<Range2>\nUpper limit for max(range 2) - min(range 2)\nnumeric\nValid Values: -256 dBpp to 256 dBpp\n\nAvailable Repeated Capabilities:\ninstance: i0, i1, i2, i3, i4, i5, i6, i7, i8, i9, i10, i11, i12, i13, i14, i15, i16, i17, i18, i19, i20, i21, i22, i23, i24, i25, i26, i27, i28, i29, i30, i31, i32\r\n\nRemote-control command(s):\nCONFigure:NRSub:MEAS<i>:MEValuation:LIMit:BPWShaping:ESFLatness"}, {"Level"=4, "Class Only"=TRUE, "Identifier"="", "Descriptive Name"="QPSK", "Data Type"=enum."ViInt32", "Command"="", "Access"=enum."Read Only", "Range Table"="", "Read Callback"="", "Write Callback"="", "Range Callback"="", "Check Callback"="", "Rngtable Callback"="", "Coerce Callback"="", "Supported Models"="", "Instrument Options"="", "Check Status Callback"="", "Flags"=0, "Help"="QPSK modulation limits definition."}, {"Level"=5, "Class Only"=FALSE, "Identifier"="RSCMWXPNRFR1M_ATTR_MULTI_EVAL_MEAS_LIMIT_QPSK_EVM", "Descriptive Name"="Multi Eval Meas Limit QPSK EVM", "Data Type"=enum."RawString", "Command"="CONF:NRS:MEAS{instance}:MEV:LIM:QPSK:EVM", "Access"=enum."Read/Write", "Range Table"="", "Read Callback"="", "Write Callback"="", "Range Callback"="", "Check Callback"="", "Rngtable Callback"="", "Coerce Callback"="", "Supported Models"="", "Instrument Options"="", "Check Status Callback"="", "Flags"=0, "Help"="Defines upper limits for the RMS and peak values of the error vector magnitude (EVM) for QPSK.\n\nSyntax:\nCONFigure:NRSub:MEAS<i>:MEValuation:LIMit:QPSK:EVMagnitude <RMS>, <Peak>\n\n<RMS>\nnumeric | ON | OFF\nValid Values:\n0 % to 100 %\n  \n<Peak>\nnumeric | ON | OFF\nValid Values:\n0 % to 100 %\n\nAvailable Repeated Capabilities:\ninstance: i0, i1, i2, i3, i4, i5, i6, i7, i8, i9, i10, i11, i12, i13, i14, i15, i16, i17, i18, i19, i20, i21, i22, i23, i24, i25, i26, i27, i28, i29, i30, i31, i32\r\n\nRemote-control command(s):\nCONFigure:NRSub:MEAS<i>:MEValuation:LIMit:QPSK:EVMagnitude"}, {"Level"=5, "Class Only"=FALSE, "Identifier"="RSCMWXPNRFR1M_ATTR_MULTI_EVAL_MEAS_LIMIT_QPSK_MERR", "Descriptive Name"="Multi Eval Meas Limit QPSK MERR", "Data Type"=enum."RawString", "Command"="CONF:NRS:MEAS{instance}:MEV:LIM:QPSK:MERR", "Access"=enum."Read/Write", "Range Table"="", "Read Callback"="", "Write Callback"="", "Range Callback"="", "Check Callback"="", "Rngtable Callback"="", "Coerce Callback"="", "Supported Models"="", "Instrument Options"="", "Check Status Callback"="", "Flags"=0, "Help"="Defines upper limits for the RMS and peak values of the magnitude error (MERR)  for QPSK.\n\nSyntax:\nCONFigure:NRSub:MEAS<i>:MEValuation:LIMit:QPSK:MERRor <RMS>, <Peak>\n\n<RMS>\nnumeric | ON | OFF\nValid Values:\n0 % to 100 %\n  \n<Peak>\nnumeric | ON | OFF\nValid Values:\n0 % to 100 %\n\nAvailable Repeated Capabilities:\ninstance: i0, i1, i2, i3, i4, i5, i6, i7, i8, i9, i10, i11, i12, i13, i14, i15, i16, i17, i18, i19, i20, i21, i22, i23, i24, i25, i26, i27, i28, i29, i30, i31, i32\r\n\nRemote-control command(s):\nCONFigure:NRSub:MEAS<i>:MEValuation:LIMit:QPSK:MERRor"}, {"Level"=5, "Class Only"=FALSE, "Identifier"="RSCMWXPNRFR1M_ATTR_MULTI_EVAL_MEAS_LIMIT_QPSK_PERR", "Descriptive Name"="Multi Eval Meas Limit QPSK PERR", "Data Type"=enum."RawString", "Command"="CONF:NRS:MEAS{instance}:MEV:LIM:QPSK:PERR", "Access"=enum."Read/Write", "Range Table"="", "Read Callback"="", "Write Callback"="", "Range Callback"="", "Check Callback"="", "Rngtable Callback"="", "Coerce Callback"="", "Supported Models"="", "Instrument Options"="", "Check Status Callback"="", "Flags"=0, "Help"="Defines symmetric limits for the RMS and peak values of the phase error for QPSK. The limit check fails if the absolute value of the measured phase error exceeds the specified values.\n\nSyntax:\nCONFigure:NRSub:MEAS<i>:MEValuation:LIMit:QPSK:PERRor <RMS>, <Peak>\n\n<RMS>\nnumeric | ON | OFF\nValid Values:\n0 % to 100 %\n  \n<Peak>\nnumeric | ON | OFF\nValid Values:\n0 % to 100 %\n\nAvailable Repeated Capabilities:\ninstance: i0, i1, i2, i3, i4, i5, i6, i7, i8, i9, i10, i11, i12, i13, i14, i15, i16, i17, i18, i19, i20, i21, i22, i23, i24, i25, i26, i27, i28, i29, i30, i31, i32\r\n\nRemote-control command(s):\nCONFigure:NRSub:MEAS<i>:MEValuation:LIMit:QPSK:PERRor"}, {"Level"=5, "Class Only"=FALSE, "Identifier"="RSCMWXPNRFR1M_ATTR_MULTI_EVAL_MEAS_LIMIT_QPSK_FERR_ENABLED", "Descriptive Name"="Multi Eval Meas Limit QPSK FERR Enabled", "Data Type"=enum."ViBoolean", "Command"="CONF:NRS:MEAS{instance}:MEV:LIM:QPSK:FERR", "Access"=enum."Read/Write", "Range Table"="", "Read Callback"="", "Write Callback"="", "Range Callback"="", "Check Callback"="", "Rngtable Callback"="", "Coerce Callback"="", "Supported Models"="", "Instrument Options"="", "Check Status Callback"="", "Flags"=0, "Help"="Defines an upper limit for the carrier frequency error (QPSK modulation).\n\nAvailable Repeated Capabilities:\ninstance: i0, i1, i2, i3, i4, i5, i6, i7, i8, i9, i10, i11, i12, i13, i14, i15, i16, i17, i18, i19, i20, i21, i22, i23, i24, i25, i26, i27, i28, i29, i30, i31, i32\r\n\nRemote-control command(s):\nCONFigure:NRSub:MEAS<i>:MEValuation:LIMit:QPSK:FERRor"}, {"Level"=5, "Class Only"=FALSE, "Identifier"="RSCMWXPNRFR1M_ATTR_MULTI_EVAL_MEAS_LIMIT_QPSK_FERR", "Descriptive Name"="Multi Eval Meas Limit QPSK FERR", "Data Type"=enum."ViReal64", "Command"="CONF:NRS:MEAS{instance}:MEV:LIM:QPSK:FERR", "Access"=enum."Read/Write", "Range Table"="rsCmwxpNrFr1M_rngFERR", "Read Callback"="", "Write Callback"="", "Range Callback"="", "Check Callback"="", "Rngtable Callback"="", "Coerce Callback"="", "Supported Models"="", "Instrument Options"="", "Check Status Callback"="", "Flags"=0, "Help"="Defines an upper limit for the carrier frequency error (QPSK modulation).\n\nAvailable Repeated Capabilities:\ninstance: i0, i1, i2, i3, i4, i5, i6, i7, i8, 
